vi "libssh2_channel_window_read_ex.vi"(8 "error in (no error)":errorcluster, 11 "channel":T1) -> (0 "error out":errorcluster, 1 "bytes available for read":u32, 2 "initial window size":u32, 3 "remaining read window":u32)   [LabVIEW 2013, in "libssh2.lvlib"]
doc: "Returns the number of bytes which the remote end may send without overflowing the window limit.\n\n<B>bytes available for read</B> returns the number of bytes actually available to be read.\n<B>initial window size</B> returns the initial window size as defined by the channel_open request."
uses:
  libssh2.lvlib
  Channel Refnum.ctl
  Not A Channel.vi
  <vilib>/Utility/error.llb/Error Cluster From Error Code.vi
  Global Settings.vi
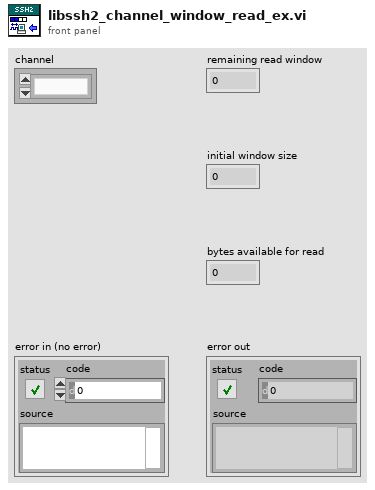
[diagram p1: front panel]
types:
  T1 = typedef "libssh2.lvlib/Channel Refnum.ctl" = refnum<k1>
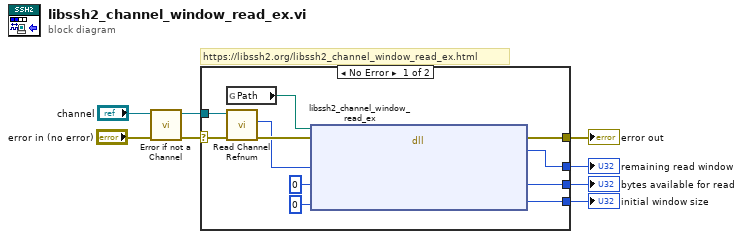
[diagram p0: block diagram]
diagram:
  # "https://libssh2.org/libssh2_channel_window_read_ex.html"
  n1 = call "Error if not a Channel.vi"("error in (no error)"="error in (no error)", "channel"="channel") -> ("error out"=w3:errorcluster, "channel out"=w1:T1)  [unwired: 8 in]
  n2 = case shown="No Error" w3 {
    selector: w3 -> [w19 w20]
    tunnel: [w18 w20] -> w8
    tunnel: w1 -> [w17 _]
    tunnel: [w16 _] -> w6
    tunnel: [w15 _] -> w5
    tunnel: [w14 _] -> w4
    frame No Error {
      n3 = global read "Global Settings.vi" "Path"() -> (w11:path)
      n4 = call "Read Channel Refnum.vi"("error in (no error)"=w19, "channel"=w17) -> ("error out"=w13:errorcluster, "LIBSSH2_CHANNEL*"=w12:u64)  [unwired: 8 in]
      n5 = dll-call lib="?" fn="libssh2_channel_window_read_ex"(path in=w11, error in=w13, "channel"=w12, "read_avail"=u32 0, "window_size_initial"=u32 0) -> (error out=w18:errorcluster, "return value"=w15:u32, "read_avail"=w14:u32, "window_size_initial"=w16:u32)  [unwired: 2 in, 1 out]
    }
    frame Error {
    }
  }
  "error out" <- w8
  "initial window size" <- w6
  "remaining read window" <- w5
  "bytes available for read" <- w4
